vi "Complex To Polar.vi"   [LabVIEW 2010, in "NI_Matrix.lvlib"]
doc: "Breaks a complex number into its polar components."
uses:
  NI_Matrix.lvlib
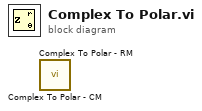
[diagram p0: block diagram]
diagram:
  n1 = call "Complex To Polar - CM.vi"() -> ()  [unwired: 1 in, 2 out]
  n2 = call "Complex To Polar - RM.vi"() -> ()  [unwired: 1 in, 2 out]
